vi "Get Control Reference.vi"(8 "error in (no error)":errorcluster, 11 "Item Configuration in":refnum<class "Item Configuration.lvclass">) -> (0 "error out":errorcluster, 2 "Control Reference":refnum<vi>, 3 "Item Configuration out":refnum<class "Item Configuration.lvclass">)   [LabVIEW 2013, in "Item Configuration.lvlib" / "Item Configuration.lvclass"]
uses:
  Item Configuration.lvclass
  Item Configuration.lvclass/Item Configuration.ctl
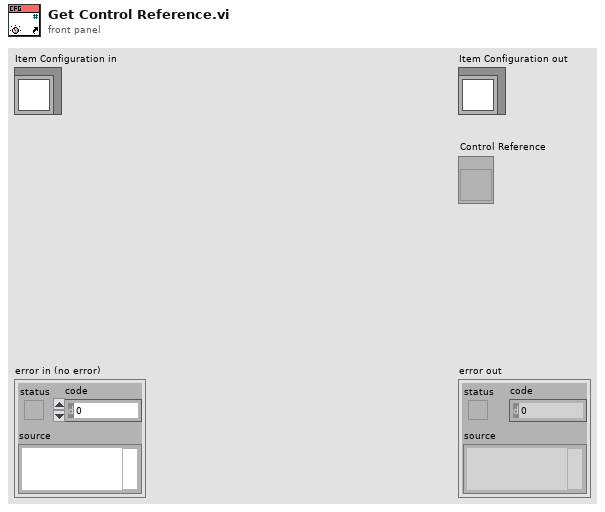
[diagram p1: front panel]
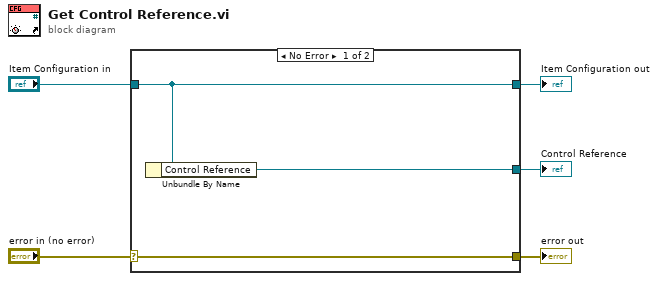
[diagram p0: block diagram]
diagram:
  n1 = case shown="No Error" "error in (no error)" {
    selector: "error in (no error)" -> [w8 w9]
    tunnel: [w8 w9] -> w4
    tunnel: [w7 w10] -> w2
    tunnel: "Item Configuration in" -> [w7 w10]
    tunnel: [w6 _] -> w1
    frame No Error {
      n2 = Unbundle By Name(w7) -> ("Control Reference"=w6:refnum<vi>)
    }
    frame Error {
    }
  }
  "error out" <- w4
  "Item Configuration out" <- w2
  "Control Reference" <- w1
